vi "Setup UI.vi"(8 "error in (no error)":errorcluster, 10 "Set UI to input? (F)":bool, 11 "Wavelength PEM and Digikröm in":refnum<class "Wavelength PEM and Digikröm.lvclass">) -> (0 "error out":errorcluster, 3 "Wavelength PEM and Digikröm out":refnum<class "Wavelength PEM and Digikröm.lvclass">)   [LabVIEW 2017, in "Wavelength PEM and Digikröm.lvclass"]
doc: "Scanner::Setup is a constructor that has no parameters and faces the user. The Factory calls this VI to let the user configure this Scanner. It is dynamically dispatched in order to let the user choose the type as well as the options of the scanner."
uses:
  Instruments/Utility Classes/Scannable/Scannable.lvclass
panel:
  in  "Inhibited":bool
  in  "Retardation":dbl
  in  "Go to first point":bool
  in  "Set Properties":bool
  out "Suggested Step Size":dbl
  in  "Exit Slit":dbl[unit]=9.999999999999999e-06
  in  "Entrance Slit":dbl[unit]=9.999999999999999e-06
  out "Ready":bool
  # "PEM and Digikrom Setup"
  # "Digikrom"
  # "PEM"
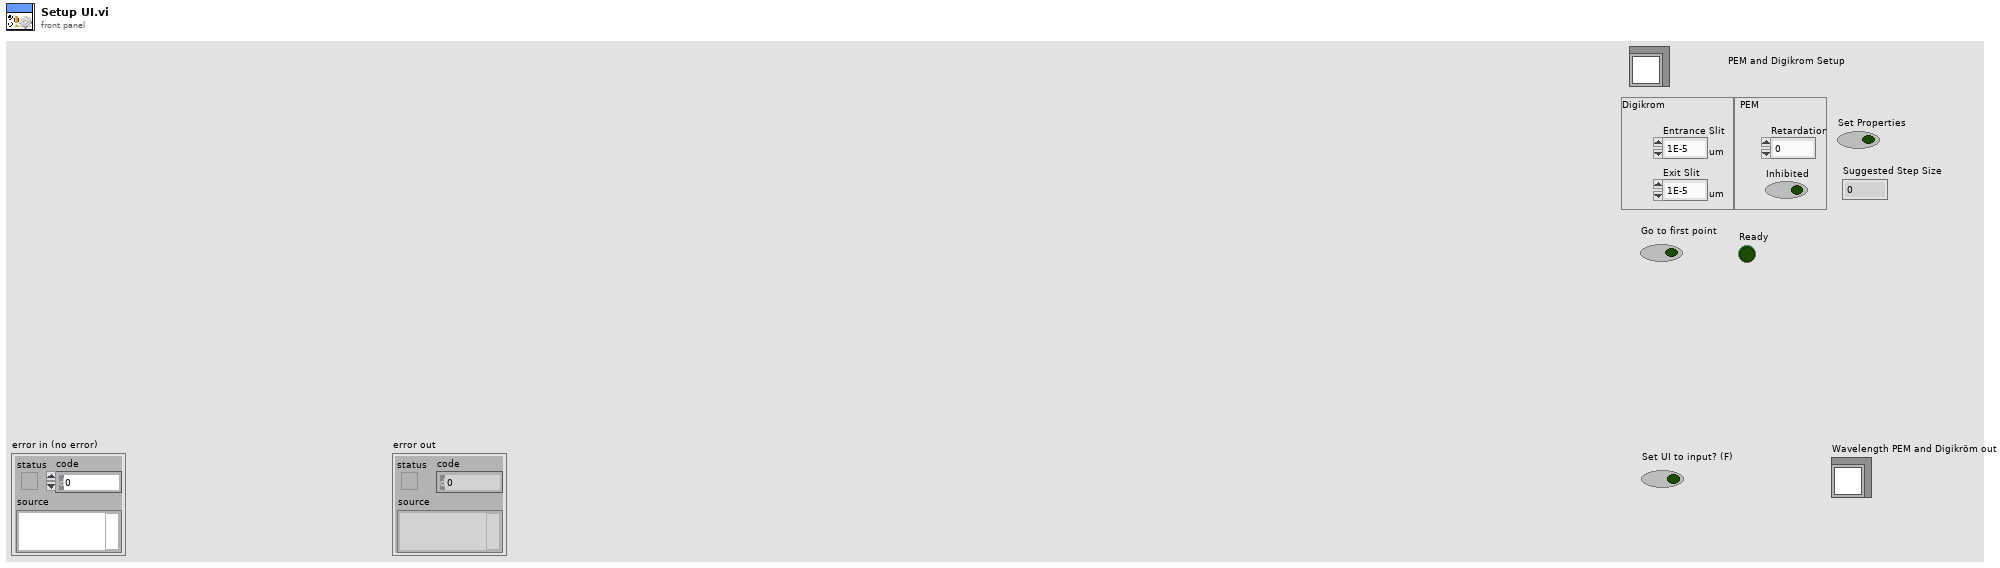
[diagram p1: front panel]
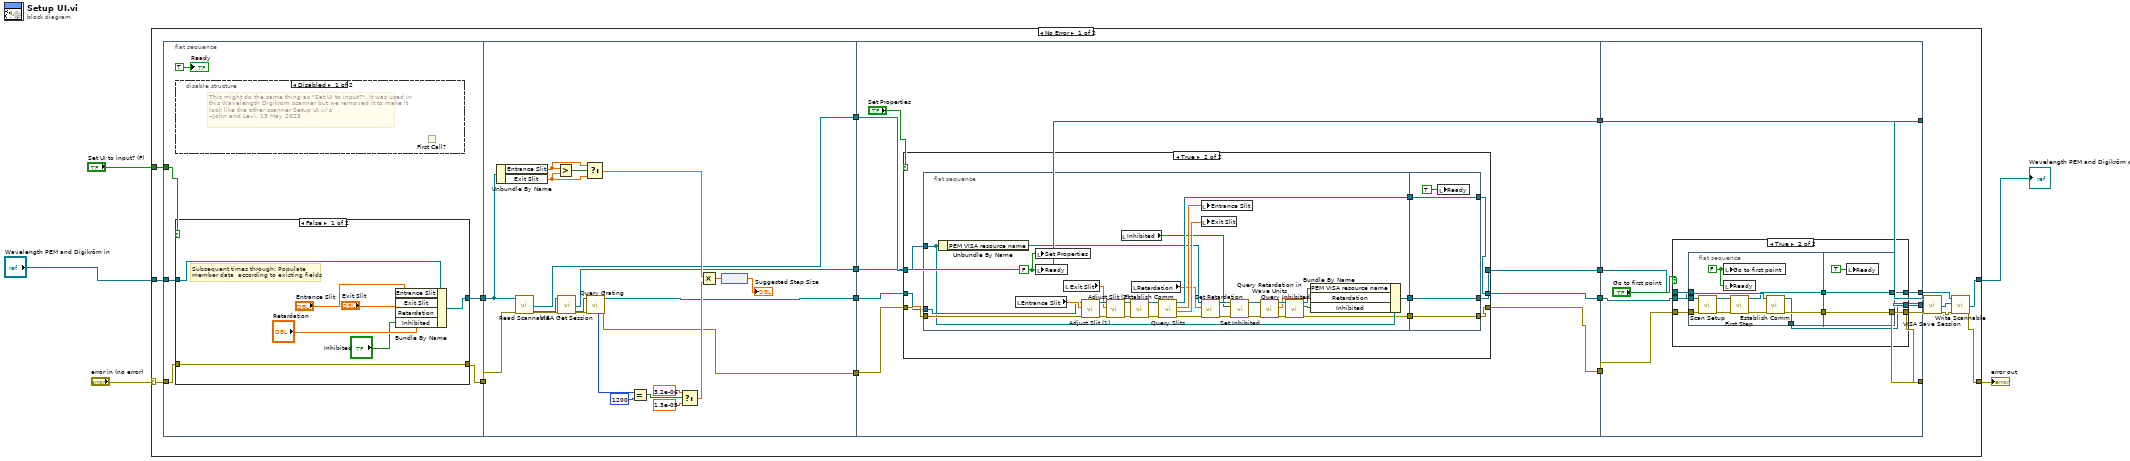
[diagram p0: block diagram]
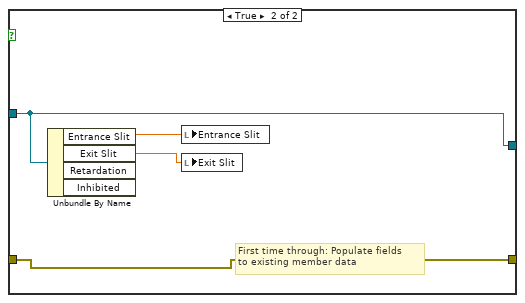
[diagram p3: hidden frame]
diagram:
  n1 = case shown="No Error" "error in (no error)" {
    selector: "error in (no error)" -> [w25 w152]
    tunnel: "Wavelength PEM and Digikröm in" -> [w26 w153]
    tunnel: "Set UI to input? (F)" -> [w20 _]
    tunnel: [w11 w152] -> w3
    tunnel: [w10 w153] -> w1
    frame No Error {
      n2 = flat-sequence {
        tunnel: w26 -> [w30]
        tunnel: [w31] -> w19
        tunnel: w25 -> [w32]
        tunnel: [w28] -> w18
        tunnel: w20 -> [w29]
        tunnel: [w47] -> w24
        tunnel: [w46] -> w22
        tunnel: w18 -> [w50]
        tunnel: w19 -> [w55]
        tunnel: [w45] -> w17
        tunnel: [w44] -> w14
        tunnel: w24 -> [w66]
        tunnel: [w73] -> w23
        tunnel: w22 -> [w71]
        tunnel: [w72] -> w21
        tunnel: w17 -> [w69]
        tunnel: [w68] -> w16
        tunnel: [w67] -> w15
        tunnel: w14 -> [w67]
        tunnel: [w123] -> w7
        tunnel: [w124] -> w8
        tunnel: w23 -> [w125]
        tunnel: w21 -> [w126]
        tunnel: w16 -> [w122]
        tunnel: [w121] -> w6
        tunnel: w15 -> [w120]
        tunnel: [w120] -> w9
        frame #0 {
          n3 = disable-structure shown="Disabled" {
            frame Disabled {
              # "This might do the same thing as \"Set UI to input?\". It was used in this Wavelength Digikrom scanner but we removed it to make it look like the other scanner Setup UI.vi's\n--John and Levi, 13 May 2023"
              n4 = First Call?() -> ()  [unwired: 1 out]
            }
            frame Enabled {
            }
          }
          n5 = case shown="False" w29 {
            tunnel: w30 -> [w38 w40]
            tunnel: w32 -> [w39 w41]
            tunnel: [w39 w41] -> w31
            tunnel: [w35 w40] -> w28
            frame False {
              # "Subsequent times through: Populate \nmember data  according to existing fields"
              n6 = Bundle By Name(cluster=w38, "Entrance Slit"="Entrance Slit", "Exit Slit"="Exit Slit", "Retardation"="Retardation", "Inhibited"="Inhibited") -> (w35:refnum<class "Wavelength PEM and Digikröm.lvclass">)
            }
            frame True {
              # "First time through: Populate fields  \nto existing member data"
              n7 = Unbundle By Name(w40) -> ("Entrance Slit"=w43:dbl[unit], "Exit Slit"=w42:dbl[unit])  [unwired: 2 out]
              n8 = local write "Entrance Slit"(w43) -> ()
              n9 = local write "Exit Slit"(w42) -> ()
            }
          }
          "Ready" <- TRUE ("Ready")
        }
        frame #1 {
          n10 = Unbundle By Name(w50) -> ("Entrance Slit"=w49:dbl[unit], "Exit Slit"=w48:dbl[unit])
          n11 = call-dynamic "Read Scannable.vi"("error in (no error)"=w55, "Scanner.lvclass in"=w50) -> ("error out"=w54:errorcluster, "Scannable.lvclass"=w52:refnum<class "Scannable.lvclass">, "Scanner.lvclass out"=w46:refnum<class "Wavelength PEM and Digikröm.lvclass">)  [unwired: 7 out]
          n12 = Greater?(x=w49, y=w48) -> (0:w65:bool)
          n13 = call-dynamic "VISA Get Session.vi"("error in (no error)"=w54, "Instrument.lvclass in"=w52) -> ("error out"=w53:errorcluster, "VISA Resource Name"=w51:refnum<visa-resource-name>, "Instrument.lvclass out"=w44:refnum<class "Scannable.lvclass">)  [unwired: 7 out]
          n14 = Select(t=w49, s=w65, f=w48) -> (s? t:f=w59:dbl[unit])
          n15 = call "Query Grating.vi"("error in (no error)"=w53, "VISA resource name"=w51) -> ("error out"=w47:errorcluster, "VISA resource name out"=w45:refnum<visa-resource-name>, "GR/MM"=w64:u16)  [unwired: 4 in, 3 out]
          n16 = Equal?(x=w64, y=u16 1200) -> (x = y?=w62:bool)
          n17 = Select(t=3.2e-06, s=w62, f=1.3e-05) -> (s? t:f=w58:dbl)
          n18 = Multiply(x=w59, y=w58) -> (x*y=w57:dbl[unit])
          n19 = node(w57) -> (→"Suggested Step Size":dbl)
        }
        frame #2 {
          n20 = case shown="True" "Set Properties" {
            tunnel: w66 -> [w76 w85]
            tunnel: [w76 w84] -> w73
            tunnel: [w75 w83] -> w72
            tunnel: w71 -> [w75 w82]
            tunnel: w69 -> [w74 w80]
            tunnel: [w74 w78] -> w68
            frame False {
            }
            frame True {
              n21 = flat-sequence {
                tunnel: w85 -> [w109]
                tunnel: w82 -> [w100]
                tunnel: [w91] -> w81
                tunnel: w80 -> [w103]
                tunnel: [w101] -> w79
                tunnel: [w102] -> w77
                tunnel: [w117] -> w83
                tunnel: [w119] -> w84
                tunnel: w81 -> [w119]
                tunnel: w79 -> [w117]
                tunnel: [w116] -> w78
                tunnel: w77 -> [w116]
                frame #0 {
                  w106 = FALSE ("Set Slits")
                  n22 = Unbundle By Name(w100) -> ("PEM VISA resource name"=w97:refnum<visa-resource-name>)
                  n23 = local read "Entrance Slit"() -> (w105:dbl[unit])
                  n24 = local write "Set Properties"(w106) -> ()
                  n25 = local write "Ready"(w106) -> ()
                  n26 = local read "Exit Slit"() -> (w104:dbl[unit])
                  n27 = call "Adjust Slit (1).vi"("error in (no error)"=w109, "SLIT WIDTH"=w105, "VISA resource name"=w103) -> ("error out"=w112:errorcluster, "VISA resource name out"=w115:refnum<visa-resource-name>)  [unwired: 7 out]
                  n28 = call "Adjust Slit (2).vi"("error in (no error)"=w112, "SLIT WIDTH"=w104, "VISA resource name"=w115) -> ("error out"=w111:errorcluster, "VISA resource name out"=w114:refnum<visa-resource-name>)  [unwired: 7 out]
                  n29 = local read "Inhibited"() -> (w95:bool)
                  n30 = call "Establish Comm.vi"("error in (no error)"=w111, "VISA resource name"=w114) -> ("error out"=w110:errorcluster, "VISA resource name out"=w113:refnum<visa-resource-name>)  [unwired: 8 in]
                  n31 = local read "Retardation"() -> (w94:dbl)
                  n32 = call "Query Slits.vi"("error in (no error)"=w110, "VISA resource name"=w113) -> ("error out"=w99:errorcluster, "CURRENT S2 WIDTH"=w107:dbl[unit], "CURRENT S1 WIDTH"=w108:dbl[unit], "VISA resource name out"=w102:refnum<visa-resource-name>)  [unwired: 6 out]
                  n33 = local write "Entrance Slit"(w108) -> ()
                  n34 = local write "Exit Slit"(w107) -> ()
                  n35 = call "Set Retardation.vi"("error in (no error)"=w99, "Retardation"=w94, "VISA resource name"=w97) -> ("error out"=w98:errorcluster, "VISA resource name out"=w96:refnum<visa-resource-name>)  [unwired: 6 in, 1 out]
                  n36 = call "Set Inhibited.vi"("error in (no error)"=w98, "Inhibit"=w95, "VISA resource name"=w96) -> ("error out"=w93:errorcluster, "VISA resource name out"=w90:refnum<visa-resource-name>)  [unwired: 6 in, 1 out]
                  n37 = call "Query Retardation in Wave Units.vi"("error in (no error)"=w93, "VISA resource name"=w90) -> ("error out"=w92:errorcluster, "Fraction of wave Retardation"=w86:dbl, "VISA resource name out"=w89:refnum<visa-resource-name>)  [unwired: 7 in]
                  n38 = call "Query Inhibited.vi"("error in (no error)"=w92, "VISA resource name"=w89) -> ("error out"=w91:errorcluster, "Inibit"=w87:bool, "VISA resource name out"=w88:refnum<visa-resource-name>)  [unwired: 7 in]
                  n39 = Bundle By Name(cluster=w100, "PEM VISA resource name"=w88, "Retardation"=w86, "Inhibited"=w87) -> (w101:refnum<class "Wavelength PEM and Digikröm.lvclass">)
                }
                frame #1 {
                  n40 = local write "Ready"(TRUE ("Ready")) -> ()
                }
              }
            }
          }
        }
        frame #3 {
          n41 = case shown="True" "Go to first point" {
            tunnel: w126 -> [w130 w137]
            tunnel: [w130 w135] -> w123
            tunnel: [w129 w136] -> w124
            tunnel: w125 -> [w129 w138]
            tunnel: w122 -> [w128 w132]
            tunnel: [w128 w131] -> w121
            frame False {
            }
            frame True {
              n42 = flat-sequence {
                tunnel: w138 -> [w148]
                tunnel: w137 -> [w147]
                tunnel: [w142] -> w134
                tunnel: [w140] -> w133
                tunnel: w132 -> [w141]
                tunnel: [w139] -> w131
                tunnel: [w150] -> w135
                tunnel: [w151] -> w136
                tunnel: w134 -> [w151]
                tunnel: w133 -> [w150]
                frame #0 {
                  w144 = FALSE ("Go to first point")
                  n43 = call-dynamic "Scan Setup.vi"("error in (no error)"=w148, "Wavelength PEM and Digikröm in"=w147) -> ("error out"=w146:errorcluster, "Wavelength PEM and Digikröm out"=w145:refnum<class "Wavelength PEM and Digikröm.lvclass">)  [unwired: 8 in]
                  n44 = local write "Go to first point"(w144) -> ()
                  n45 = local write "Ready"(w144) -> ()
                  n46 = call-dynamic "First Step.vi"("error in (no error)"=w146, "Wavelength PEM and Digikröm.lvclass in"=w145) -> ("error out"=w143:errorcluster, "Wavelength PEM and Digikröm.lvclass out"=w140:refnum<class "Wavelength PEM and Digikröm.lvclass">)  [unwired: 7 in, 1 out]
                  n47 = call "Establish Comm.vi"("error in (no error)"=w143, "VISA resource name"=w141) -> ("error out"=w142:errorcluster, "VISA resource name out"=w139:refnum<visa-resource-name>)  [unwired: 8 in]
                }
                frame #1 {
                  n48 = local write "Ready"(TRUE ("Ready")) -> ()
                }
              }
            }
          }
        }
      }
      n49 = call-dynamic "VISA Save Session.vi"("error in (no error)"=w8, "VISA Resource Name"=w6, "Instrument.lvclass in"=w9) -> ("error out"=w12:errorcluster, "Instrument.lvclass out"=w13:refnum<class "Scannable.lvclass">)  [unwired: 7 out]
      n50 = call-dynamic "Write Scannable.vi"("error in (no error)"=w12, "Scannable.lvclass"=w13, "Scanner.lvclass in"=w7) -> ("error out"=w11:errorcluster, "Scanner.lvclass out"=w10:refnum<class "Wavelength PEM and Digikröm.lvclass">)  [unwired: 7 out]
    }
    frame Error {
    }
  }
  "error out" <- w3
  "Wavelength PEM and Digikröm out" <- w1
